vi "read version information.vi"(11 "Builder in":refnum<class "Builder.lvclass">) -> (2 "version information":T1)   [LabVIEW 2024, in "Builder.lvclass"]
uses:
  Builder.lvclass
  Builder.lvclass/Builder.ctl
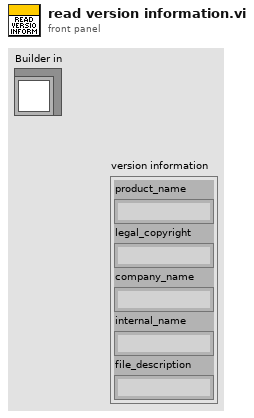
[diagram p1: front panel]
types:
  T1 = cluster{"product_name":string, "legal_copyright":string, "company_name":string, "internal_name":string, "file_description":string}
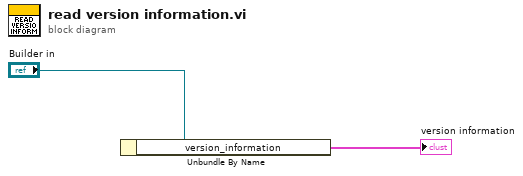
[diagram p0: block diagram]
diagram:
  n1 = Unbundle By Name("Builder in") -> ("version_information"=→"version information":T1)
